vi "Ch_data_pattern_4_save (SubVI).vi"(7 "error in":errorcluster, 14 "T Cluster":cluster{"T1":dbl, "T2":dbl, "T3":dbl, "T4":dbl}, 15 "Activate!":bool, 17 "file":refnum<file>) -> (27 "error out":errorcluster)   [LabVIEW 2015]
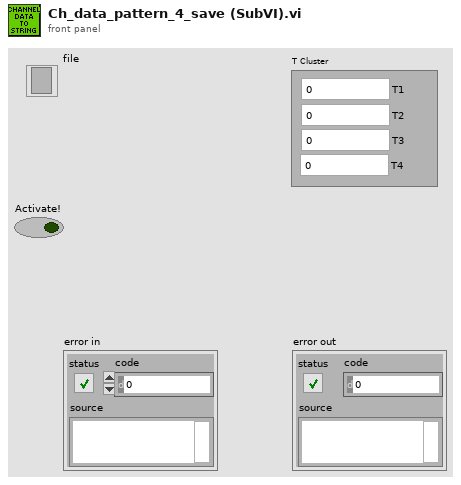
[diagram p1: front panel]
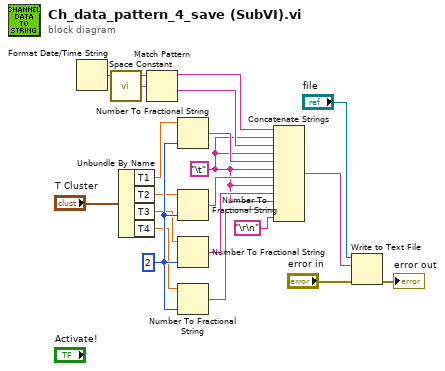
[diagram p0: block diagram]
diagram:
  w7 = i16 2 ("precision (6)")
  w8 = "\t"
  n1 = Format Date/Time String() -> (date/time string=w18:string)  [unwired: 3 out]
  n2 = call <vilib>:"Space Constant.vi"() -> ("String"=w19:string)
  n3 = Unbundle By Name("T Cluster") -> ("T1"=w5:dbl, "T2"=w4:dbl, "T3"=w3:dbl, "T4"=w2:dbl)
  n4 = Match Pattern(string=w18, regular expression=w19) -> (before substring=w11:string, after substring=w10:string)  [unwired: 3 out]
  n5 = Number To Fractional String(number=w5, precision (6)=w7) -> (F-format string=w16:string)  [unwired: 2 out]
  n6 = Number To Fractional String(number=w4, precision (6)=w7) -> (F-format string=w12:string)  [unwired: 2 out]
  n7 = Number To Fractional String(number=w3, precision (6)=w7) -> (F-format string=w15:string)  [unwired: 2 out]
  n8 = Number To Fractional String(number=w2, precision (6)=w7) -> (F-format string=w14:string)  [unwired: 2 out]
  n9 = Concatenate Strings(w11, w8, w10, w8, w16, w8, w12, w8, w15, w8, w14, "\r\n") -> (w9:string)
  n10 = Write to Text File(file (use dialog)="file", text=w9, error in="error in") -> (error out=→"error out":errorcluster)  [unwired: 3 out]
